vi "CML Main.vi"() -> ()   [LabVIEW 2024]
doc: "This Continuous Measurement sample project is based on the Queued Message Handler template.\n\nThe Event Handling Loop generates messages based on user interface actions.\n\nThe Message Handling Loop processes messages generated by the Event Handling Loop, or by other messages. There are also Acquisition and Logging message handling loop subVIs, and a chart updating loop."
uses:
  Settings/Settings.ctl
  Acquisition/Hardware Configuration.ctl
  Acquisition/Signal Type.ctl
  Logging/Logging Configuration.ctl
  controls/CML UI Data.ctl
  controls/CML UI State.ctl
  Logging/Logging State.ctl
  Acquisition/Acquisition State.ctl
  support/Message Queue/Enqueue Message (Single).vi
  <vilib>/Utility/error.llb/Error Cluster From Error Code.vi
  support/Message Queue/Enqueue Message (Array).vi
  <vilib>/ErrorRing/Error Ring.xnode
  Settings/CML Settings.lvlib
  Acquisition/CML Acquisition.lvlib
  Logging/CML Logging.lvlib
  support/User Event - Stop/CML User Event - Stop.lvlib
  support/Message Queue/CML Message Queue.lvlib
  Settings/Settings Dialog.vi
panel:
  out "Data":waveform(dbl)[](graph)
  in  "Settings":bool
  in  "Start":bool
  in  "Stop":bool
  out "Status":string
  in  "Exit":bool
  # "Continuous Measurement Data Logger"
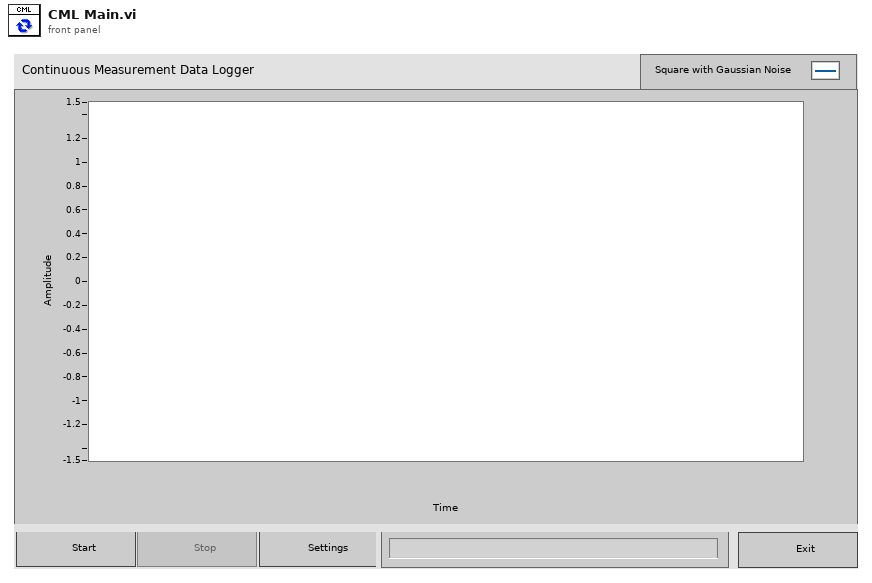
[diagram p1: front panel]
types:
  T1 = typedef "CML UI State.ctl" = enum16{"Idle", "Acquiring and Logging", "Waiting for Exit", "Waiting for Exit (Acq Stopped)", "Waiting for Exit (Log Stopped)", "Waiting for Stop", "Waiting for Stop (Acq Stopped)", "Waiting for Stop (Log Stopped)"}
  T2 = typedef "CML UI Data.ctl" = cluster{"Start Ref":refnum<vi>, "Stop Ref":refnum<vi>, "Settings Ref":refnum<vi>, "Exit Ref":refnum<vi>, "Status Ref":refnum<vi>, "Data Ref":refnum<vi>}
  T3 = typedef "CML Settings.lvlib/Settings.ctl" = cluster{"Hardware Configuration":T4, "Logging Configuration":T6}
  T4 = typedef "CML Acquisition.lvlib/Hardware Configuration.ctl" = cluster{"HW Refnum <Replace Me>":string, "Signal Type <Replace Me>":T5}
  T5 = typedef "CML Acquisition.lvlib/Signal Type.ctl" = enum16{"Sine Wave", "Square with Noise"}
  T6 = typedef "CML Logging.lvlib/Logging Configuration.ctl" = cluster{"Log File Base Path":path, "TDMS File Reference":refnum<k34>}
  T7 = typedef "CML Message Queue.lvlib/All Message Queues.ctl" = cluster{"UI":refnum<queue>, "Acquisition":refnum<queue>, "Logging":refnum<queue>}
  T8 = typedef "CML Acquisition.lvlib/Acquisition State.ctl" = enum16{"Idle", "Acquiring"}
  T9 = typedef "CML Logging.lvlib/Logging State.ctl" = enum16{"Idle", "Logging"}
  T10 = enum16{"open", "open or create", "create or replace", "create", "open (read-only)"}
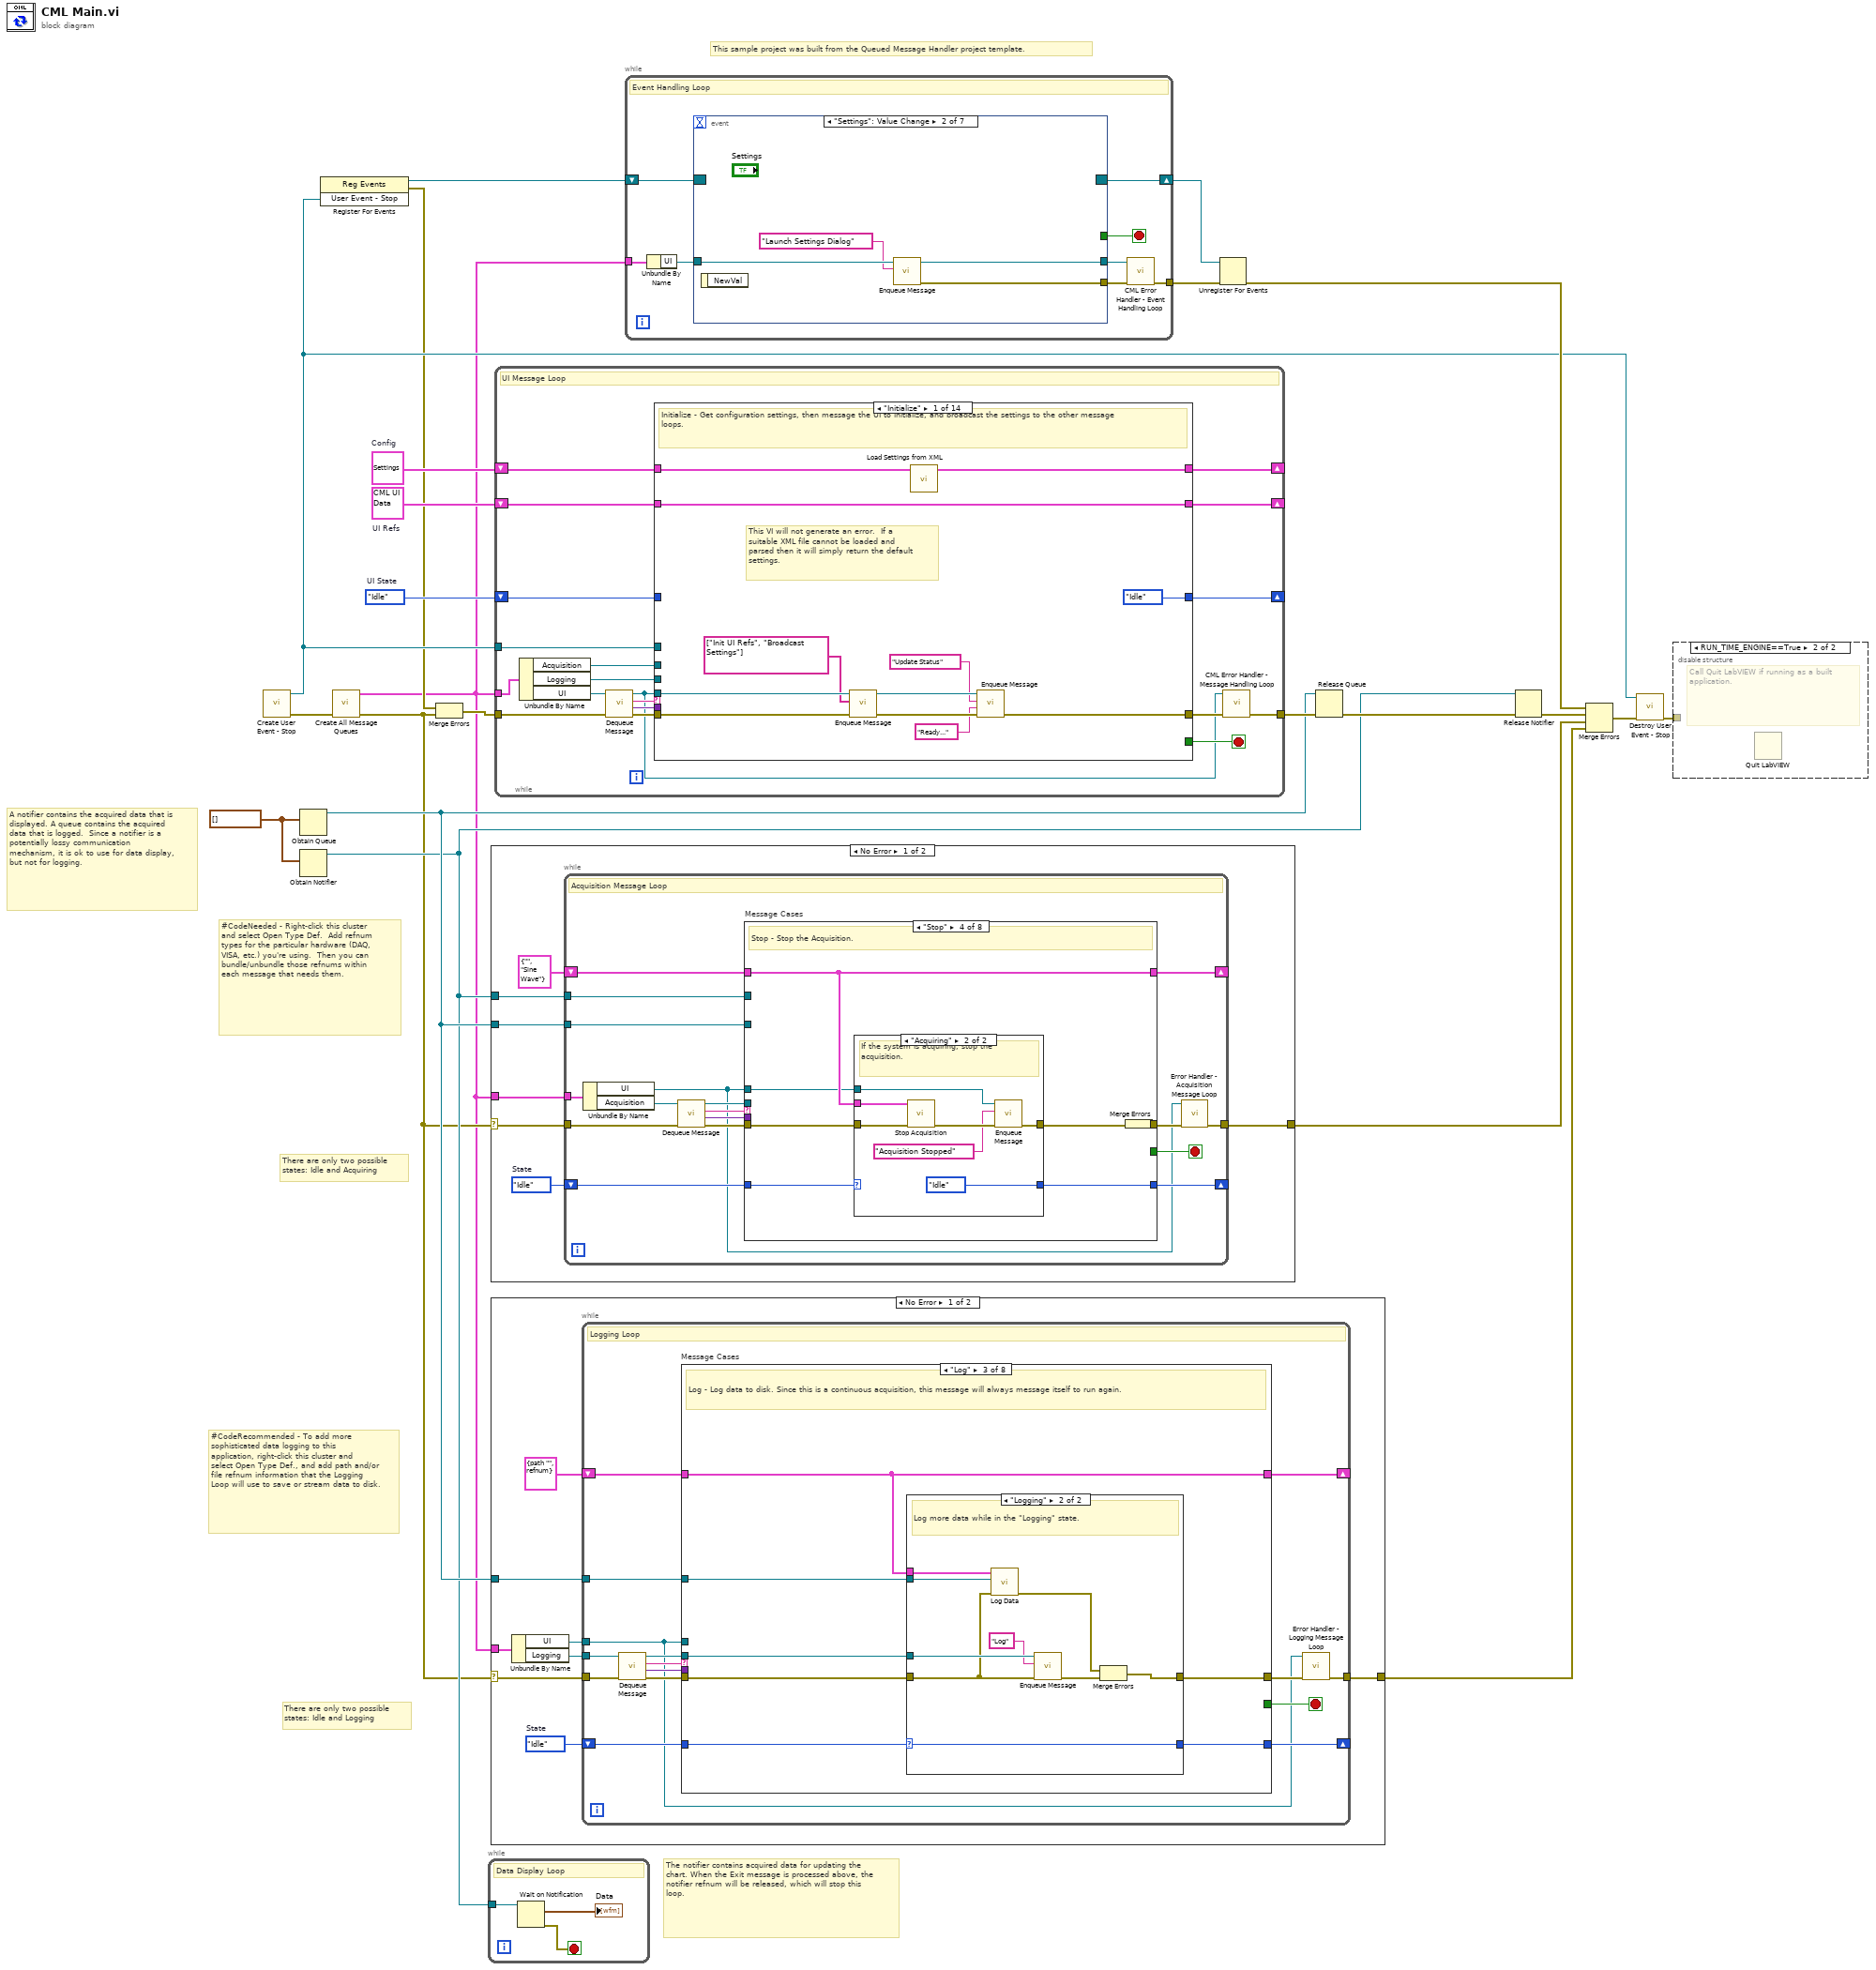
[diagram p0: block diagram]
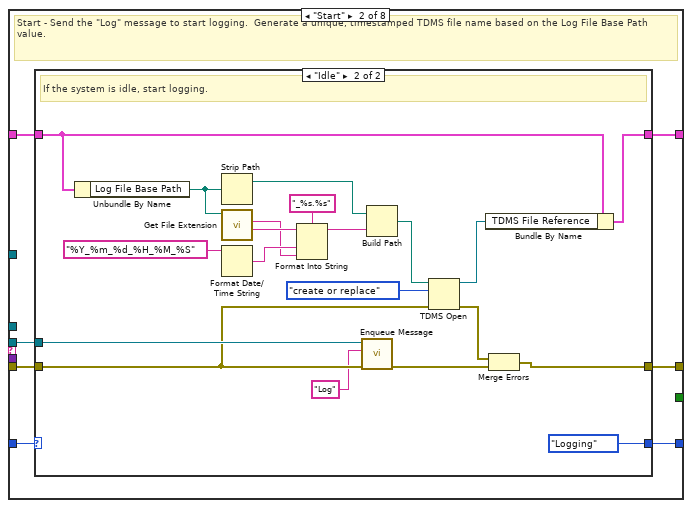
[diagram p3: hidden frame]
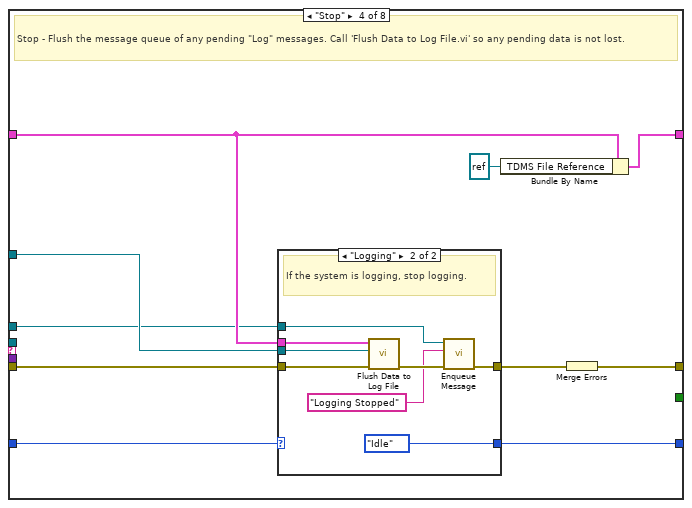
[diagram p6: hidden frame]
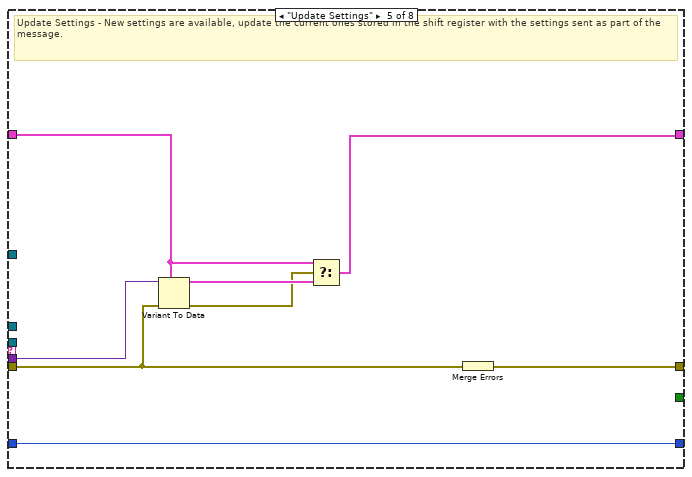
[diagram p8: hidden frame]
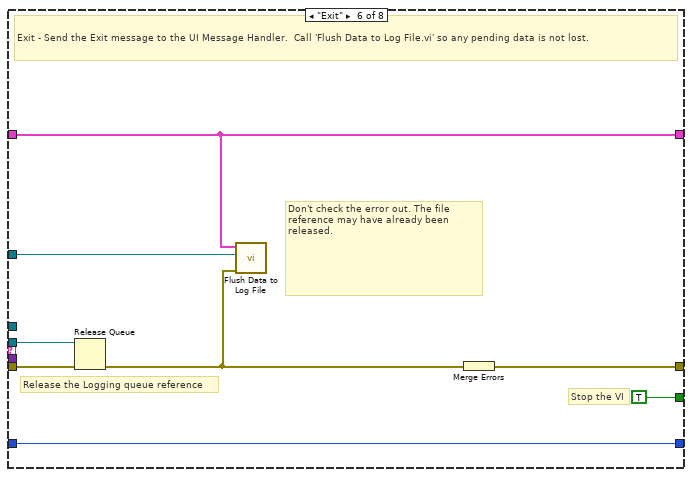
[diagram p9: hidden frame]
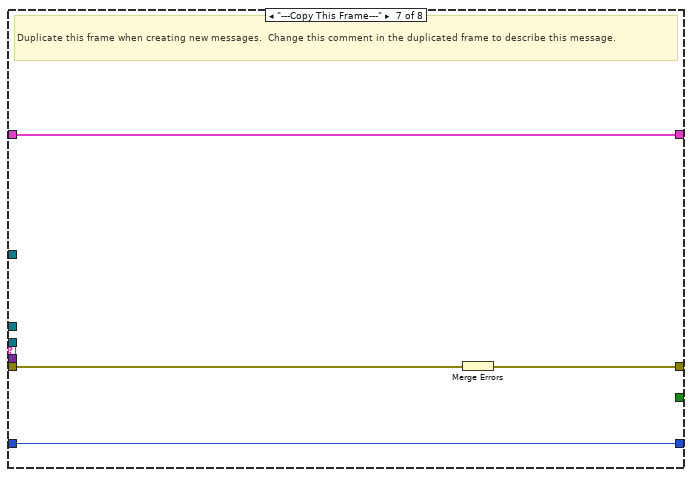
[diagram p10: hidden frame]
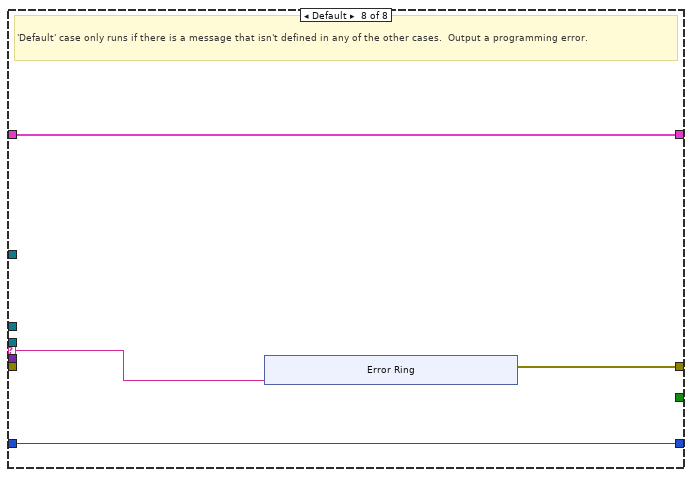
[diagram p11: hidden frame]
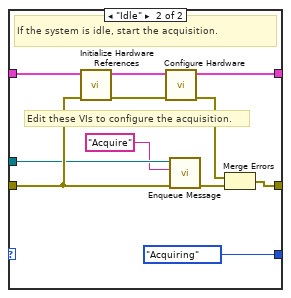
[diagram p15: hidden frame]
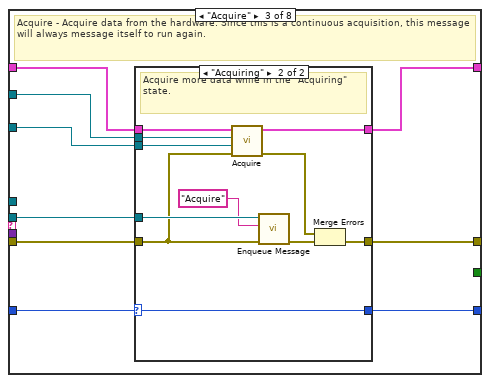
[diagram p16: hidden frame]
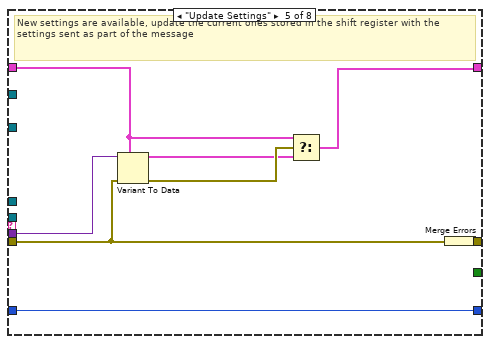
[diagram p19: hidden frame]
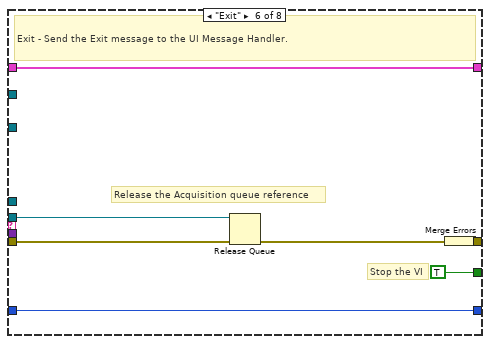
[diagram p20: hidden frame]
diagram:
  w15 = CML_UI_State."Idle"  # UI State
  w10 = waveform(dbl)[] []
  w16 = T2 {"Start Ref"=refnum, "Stop Ref"=refnum, "Settings Ref"=refnum, "Exit Ref"=refnum, "Status Ref"=refnum, "Data Ref"=refnum}  # UI Refs
  w19 = T3 {"Hardware Configuration"={"HW Refnum <Replace Me>"="", "Signal Type <Replace Me>"=enum."Sine Wave"}, "Logging Configuration"={"Log File Base Path"=path "", "TDMS File Reference"=refnum}}  # Config
  # "There are only two possible\nstates: Idle and Logging"
  # "There are only two possible\nstates: Idle and Acquiring"
  # "#CodeRecommended - To add more sophisticated data logging to this application, right-click this cluster and select Open Type Def., and add path and/or file refnum information that the Logging Loop will use to save or stream data to disk."
  # "#CodeNeeded - Right-click this cluster and select Open Type Def.  Add refnum types for the particular hardware (DAQ, VISA, etc.) you're using.  Then you can bundle/unbundle those refnums within each message that needs them."
  # "This sample project was built from the Queued Message Handler project template."
  # "A notifier contains the acquired data that is displayed. A queue contains the acquired data that is logged.  Since a notifier is a potentially lossy communication mechanism, it is ok to use for data display, but not for logging."
  # "The notifier contains acquired data for updating the chart. When the Exit message is processed above, the notifier refnum will be released, which will stop this loop."
  n1 = call "Create User Event - Stop.vi"() -> ("error out"=w20:errorcluster, "User Event - Stop"=w8:refnum<user-event>)  [unwired: 10 in]
  n2 = Obtain Queue(element data type=w10) -> (queue out=w22:refnum<queue>)  [unwired: 4 in, 2 out]
  n3 = Obtain Notifier(notification data type=w10) -> (notifier out=w5:refnum<notifier>)  [unwired: 3 in, 2 out]
  n4 = register-events(w8) -> (reference out=w9:refnum<event-registration>, error out=w6:errorcluster)  [unwired: 2 in]
  n5 = call "Create All Message Queues.vi"("error in (no error)"=w20) -> ("error out"=w3:errorcluster, "Message Queues out"=w1:T7)  [unwired: 9 in]
  n6 = Merge Errors(w6, w3) -> (w7:errorcluster)
  n7 = while "Data Display Loop" {
    tunnel: w5 -> [w26]
    stop <- w24 stop-if-true
    # "Data Display Loop"
    n8 = Wait on Notification(notifier=w26) -> (notification=→"Data":waveform(dbl)[], error out=w24:errorcluster)  [unwired: 3 in, 2 out]
  }
  n9 = case shown="No Error" w3 {
    selector: w3 -> [w31 w144]
    tunnel: w1 -> [w27 _]
    tunnel: [w33 w144] -> w4
    tunnel: w5 -> [w30 _]
    tunnel: w22 -> [w29 _]
    frame No Error {
      w28 = Acquisition_State."Idle"  # State
      n10 = while {
        shift-right: [w49] -> _
        shift-left: T4 {"HW Refnum <Replace Me>"="", "Signal Type <Replace Me>"=enum."Sine Wave"} ("Data Cluster") -> [w50]
        tunnel: w30 -> [w43]
        tunnel: w29 -> [w42]
        shift-right: [w40] -> _
        shift-left: w28 -> [w41]
        tunnel: w31 -> [w47]
        tunnel: [w39] -> w33
        tunnel: w27 -> [w36]
        stop <- w48 stop-if-true
        # "Acquisition Message Loop"
        n11 = Unbundle By Name(w36) -> ("UI"=w35:refnum<queue>, "Acquisition"=w34:refnum<queue>)
        n12 = call "Dequeue Message.vi"("error in (no error)"=w47, "Message Queue"=w34) -> ("error out"=w46:errorcluster, "Message Data"=w44:variant, "Message"=w45:string, "dup Message Queue"=w37:refnum<queue>)  [unwired: 6 in]
        n13 = case "Message Cases" shown="\"Stop\"" w45 {
          selector: w45 -> [_ _ _ _ _ _ _ w133]
          tunnel: w37 -> [_ w57 w82 _ _ w123 _ _]
          tunnel: w46 -> [w53 w58 w81 w103 w115 w125 w132 _]
          tunnel: [w53 w60 w83 w104 w121 w127 w130 w134] -> w38
          tunnel: w50 -> [w52 w59 w79 w101 w117 w126 w131 w136]
          tunnel: [w52 w56 w80 w101 w116 w126 w131 w136] -> w49
          tunnel: [_ _ _ _ _ TRUE _ _] -> w48
          tunnel: w44 -> [_ _ _ _ w120 _ _ _]
          tunnel: w35 -> [_ _ _ w98 _ _ _ _]
          tunnel: w43 -> [_ _ w78 _ _ _ _ _]
          tunnel: w42 -> [_ _ w77 _ _ _ _ _]
          tunnel: w41 -> [w51 w54 w75 w100 w114 w122 w129 w135]
          tunnel: [w51 w55 w76 w99 w114 w122 w129 w135] -> w40
          frame "Initialize" {
            # "Initialize  - Initialize is currently a no-op.  The hardware initialization takes place in the 'Start' message."
          }
          frame "Start" {
            # "Start - Configure and start the acquisition."
            n14 = case shown="\"Acquiring\"" w54 {
              selector: w54 -> [w61 _]
              tunnel: [w62 w74] -> w60
              tunnel: w59 -> [w63 w73]
              tunnel: w58 -> [w62 w72]
              tunnel: w57 -> [_ w70]
              tunnel: [w63 w66] -> w56
              tunnel: [w61 Acquisition_State."Acquiring" ("Acquisition State")] -> w55
              frame "Acquiring" {
                # "The system is already acquiring. Ignore the \"Start\" message."
              }
              frame "Idle" {
                # "Edit these VIs to configure the acquisition."
                # "If the system is idle, start the acquisition."
                n15 = call "Initialize Hardware References.vi"("error in (no error)"=w72, "Hardware Resources in"=w73) -> ("error out"=w69:errorcluster, "Hardware Resources out"=w67:T4)  [unwired: 8 in]
                n16 = call "Configure Hardware.vi"("error in (no error)"=w69, "Hardware Resources in"=w67) -> ("error out"=w68:errorcluster, "Hardware Resources out"=w66:T4)  [unwired: 8 in]
                n17 = call-poly "Enqueue Message.vi"("error in (no error)"=w72, "Message"="Acquire", "Message Queue"=w70) -> ("error out"=w71:errorcluster)  [unwired: 7 in, 1 out]
                n18 = Merge Errors(w68, w71) -> (w74:errorcluster)
              }
            }
          }
          frame "Acquire" {
            # "Acquire - Acquire data from the hardware. Since this is a continuous acquisition, this message will always message itself to run again."
            n19 = case shown="\"Acquiring\"" w75 {
              selector: w75 -> [w84 w88]
              tunnel: [w85 w97] -> w83
              tunnel: w82 -> [_ w95]
              tunnel: w81 -> [w85 w87]
              tunnel: [w86 w93] -> w80
              tunnel: w79 -> [w86 w92]
              tunnel: w78 -> [_ w90]
              tunnel: w77 -> [_ w89]
              tunnel: [w84 w88] -> w76
              frame "Idle" {
                # "Ignore \"Acquire\" messages when the acquisition is idle."
              }
              frame "Acquiring" {
                # "Acquire more data while in the \"Acquiring\" state."
                n20 = call "Acquire.vi"("error in (no error)"=w87, "Data Queue"=w89, "Data Notifier"=w90, "Hardware Resources in"=w92) -> ("error out"=w94:errorcluster, "Hardware Resources out"=w93:T4)  [unwired: 6 in]
                n21 = call-poly "Enqueue Message.vi"("error in (no error)"=w87, "Message"="Acquire", "Message Queue"=w95) -> ("error out"=w96:errorcluster)  [unwired: 7 in, 1 out]
                n22 = Merge Errors(w94, w96) -> (w97:errorcluster)
              }
            }
          }
          frame "Stop" {
            # "Stop - Stop the Acquisition."
            n23 = case shown="\"Acquiring\"" w100 {
              selector: w100 -> [w105 _]
              tunnel: w103 -> [w106 w113]
              tunnel: [w106 w109] -> w102
              tunnel: w101 -> [_ w111]
              tunnel: [w105 Acquisition_State."Idle" ("State")] -> w99
              tunnel: w98 -> [_ w108]
              frame "Idle" {
                # "The system is already idle. Ignore the \"Stop\" message."
              }
              frame "Acquiring" {
                # "If the system is acquiring, stop the acquisition."
                n24 = call "Stop Acquisition.vi"("error in (no error)"=w113, "Hardware Resources in"=w111) -> ("error out"=w112:errorcluster)  [unwired: 9 in]
                n25 = call-poly "Enqueue Message.vi"("error in (no error)"=w112, "Message"="Acquisition Stopped", "Message Queue"=w108) -> ("error out"=w109:errorcluster)  [unwired: 7 in, 1 out]
              }
            }
            n26 = Merge Errors(w102) -> (w104:errorcluster)
          }
          frame "Update Settings" {
            # "New settings are available, update the current ones stored in the shift register with the settings sent as part of the message"
            n27 = Variant To Data(error in=w115, type=w117, Variant=w120) -> (data=w118:T4, error out=w119:errorcluster)
            n28 = Select(t=w117, s=w119, f=w118) -> (s? t:f=w116:T4)
            n29 = Merge Errors(w115) -> (w121:errorcluster)
          }
          frame "Exit" {
            # "Release the Acquisition queue reference"
            # "Stop the VI"
            # "Exit - Send the Exit message to the UI Message Handler."
            n30 = Release Queue(queue=w123, error in (no error)=w125) -> (error out=w124:errorcluster)  [unwired: 1 in, 2 out]
            n31 = Merge Errors(w124) -> (w127:errorcluster)
          }
          frame "---Copy This Frame---" {
            # "Duplicate this frame when creating new messages.  Change this comment in the duplicated frame to describe this message."
            n32 = Merge Errors(w132) -> (w130:errorcluster)
          }
          frame Default {
            # "'Default' case only runs if there is a message that isn't defined in any of the other cases.  Output a programming error."
            n33 = xnode "Error Ring"("parameter 0"=w133) -> ("error out"=w134:errorcluster)
          }
        }
        n34 = call "Error Handler - Acquisition Message Loop.vi"("error in (no error)"=w38, "Message Queue"=w35) -> ("dup error in"=w39:errorcluster)  [unwired: 8 in, 1 out]
      }
    }
    frame Error {
    }
  }
  n35 = case shown="No Error" w3 {
    selector: w3 -> [w148 w270]
    tunnel: w1 -> [w152 _]
    tunnel: [w150 w270] -> w2
    tunnel: w22 -> [w147 _]
    frame No Error {
      w145 = Logging_State."Idle"  # State
      n36 = Unbundle By Name(w152) -> ("UI"=w146:refnum<queue>, "Logging"=w151:refnum<queue>)
      n37 = while {
        tunnel: w151 -> [w159]
        shift-right: [w166] -> _
        shift-left: T6 {"Log File Base Path"=path "", "TDMS File Reference"=refnum} ("Logging Configuration") -> [w167]
        tunnel: w146 -> [w153]
        tunnel: w147 -> [w158]
        shift-right: [w156] -> _
        shift-left: w145 -> [w157]
        tunnel: w148 -> [w164]
        tunnel: [w155] -> w150
        stop <- w165 stop-if-true
        # "Logging Loop"
        n38 = call "Dequeue Message.vi"("error in (no error)"=w164, "Message Queue"=w159) -> ("error out"=w163:errorcluster, "Message Data"=w161:variant, "Message"=w162:string, "dup Message Queue"=w160:refnum<queue>)  [unwired: 6 in]
        n39 = case "Message Cases" shown="\"Log\"" w162 {
          selector: w162 -> [_ _ _ _ _ _ _ w259]
          tunnel: w160 -> [_ w176 w206 _ _ w251 _ _]
          tunnel: w163 -> [w169 w175 w204 w222 w240 w252 w258 _]
          tunnel: [w169 w177 w207 w228 w246 w253 w256 w260] -> w154
          tunnel: w167 -> [w170 w174 w203 w223 w244 w249 w257 w262]
          tunnel: [w170 w173 w203 w226 w241 w249 w257 w262] -> w166
          tunnel: [_ _ _ _ _ TRUE _ _] -> w165
          tunnel: w161 -> [_ _ _ _ w245 _ _ _]
          tunnel: w153 -> [_ _ _ w219 _ _ _ _]
          tunnel: w158 -> [_ _ w205 w224 _ w248 _ _]
          tunnel: w157 -> [w168 w172 w202 w221 w239 w247 w255 w261]
          tunnel: [w168 w171 w201 w220 w239 w247 w255 w261] -> w156
          frame "Initialize" {
            # "Initialize - gets called when first launched. Currently a no-op."
          }
          frame "Start" {
            # "Start - Send the \"Log\" message to start logging.  Generate a unique, timestamped TDMS file name based on the Log File Base Path value."
            n40 = case shown="\"Idle\"" w172 {
              selector: w172 -> [w179 _]
              tunnel: [w178 w183] -> w177
              tunnel: w176 -> [_ w184]
              tunnel: w175 -> [w178 w182]
              tunnel: w174 -> [w180 w185]
              tunnel: [w180 w187] -> w173
              tunnel: [w179 Logging_State."Logging" ("State")] -> w171
              frame "Logging" {
                # "The system is already logging. Ignore the \"Start\" message."
              }
              frame "Idle" {
                # "If the system is idle, start logging."
                n41 = Unbundle By Name(w185) -> ("Log File Base Path"=w200:path)
                n42 = Strip Path(path=w200) -> (stripped path=w197:path)  [unwired: 1 out]
                n43 = call <vilib>:"Get File Extension.vi"("file"=w200) -> ("filename without extension"=w198:string, "lowercase file extension"=w194:string)  [unwired: 6 in, 3 out]
                n44 = Format Date/Time String(time format string (%c)="%Y_%m_%d_%H_%M_%S") -> (date/time string=w195:string)  [unwired: 2 in]
                n45 = Format Into String(format string="_%s.%s", initial string=w198, w195, w194) -> (resulting string=w193:string)  [unwired: 1 in, 1 out]
                n46 = call-poly "Enqueue Message.vi"("error in (no error)"=w182, "Message"="Log", "Message Queue"=w184) -> ("error out"=w190:errorcluster)  [unwired: 7 in, 1 out]
                n47 = Build Path(base path=w197, name or relative path=w193) -> (appended path=w192:path)
                n48 = TDMS Open(8:w182, 10:T10."create or replace" ("operation (0:open)"), 11:w192) -> (0:w191:errorcluster, 3:w188:refnum<k34>)  [unwired: 4 in]
                n49 = Bundle By Name(cluster=w185, "TDMS File Reference"=w188) -> (w187:T6)
                n50 = Merge Errors(w191, w190) -> (w183:errorcluster)
              }
            }
          }
          frame "Log" {
            # "Log - Log data to disk. Since this is a continuous acquisition, this message will always message itself to run again."
            n51 = case shown="\"Logging\"" w202 {
              selector: w202 -> [w209 w211]
              tunnel: [w208 w218] -> w207
              tunnel: w206 -> [_ w216]
              tunnel: w205 -> [_ w215]
              tunnel: w204 -> [w208 w210]
              tunnel: w203 -> [_ w212]
              tunnel: [w209 w211] -> w201
              frame "Idle" {
                # "Ignore \"Log\" messages when the logging is idle."
              }
              frame "Logging" {
                # "Log more data while in the \"Logging\" state."
                n52 = call "Log Data.vi"("error in (no error)"=w210, "Data Queue"=w215, "Logging Configuration"=w212) -> ("error out"=w214:errorcluster)  [unwired: 8 in]
                n53 = call-poly "Enqueue Message.vi"("error in (no error)"=w210, "Message"="Log", "Message Queue"=w216) -> ("error out"=w217:errorcluster)  [unwired: 7 in, 1 out]
                n54 = Merge Errors(w214, w217) -> (w218:errorcluster)
              }
            }
          }
          frame "Stop" {
            # "Stop - Flush the message queue of any pending \"Log\" messages. Call 'Flush Data to Log File.vi' so any pending data is not lost."
            n55 = case shown="\"Logging\"" w221 {
              selector: w221 -> [w229 _]
              tunnel: [w230 w233] -> w227
              tunnel: w224 -> [_ w237]
              tunnel: w223 -> [_ w236]
              tunnel: w222 -> [w230 w235]
              tunnel: [w229 Logging_State."Idle" ("State")] -> w220
              tunnel: w219 -> [_ w232]
              frame "Idle" {
                # "The system is already idle. Ignore the \"Stop\" message."
              }
              frame "Logging" {
                # "If the system is logging, stop logging."
                n56 = call "Flush Data to Log File.vi"("error in (no error)"=w235, "Data Queue"=w237, "Logging Configuration"=w236) -> ("error out"=w238:errorcluster)  [unwired: 8 in]
                n57 = call-poly "Enqueue Message.vi"("error in (no error)"=w238, "Message"="Logging Stopped", "Message Queue"=w232) -> ("error out"=w233:errorcluster)  [unwired: 7 in, 1 out]
              }
            }
            n58 = Bundle By Name(cluster=w223, "TDMS File Reference"=refnum<k34> refnum) -> (w226:T6)
            n59 = Merge Errors(w227) -> (w228:errorcluster)
          }
          frame "Update Settings" {
            # "Update Settings - New settings are available, update the current ones stored in the shift register with the settings sent as part of the message."
            n60 = Variant To Data(error in=w240, type=w244, Variant=w245) -> (data=w243:T6, error out=w242:errorcluster)
            n61 = Select(t=w244, s=w242, f=w243) -> (s? t:f=w241:T6)
            n62 = Merge Errors(w240) -> (w246:errorcluster)
          }
          frame "Exit" {
            # "Don't check the error out. The file reference may have already been released."
            # "Release the Logging queue reference"
            # "Stop the VI"
            # "Exit - Send the Exit message to the UI Message Handler.  Call 'Flush Data to Log File.vi' so any pending data is not lost."
            n63 = Release Queue(queue=w251, error in (no error)=w252) -> (error out=w250:errorcluster)  [unwired: 1 in, 2 out]
            n64 = call "Flush Data to Log File.vi"("error in (no error)"=w250, "Data Queue"=w248, "Logging Configuration"=w249) -> ()  [unwired: 8 in, 1 out]
            n65 = Merge Errors(w250) -> (w253:errorcluster)
          }
          frame "---Copy This Frame---" {
            # "Duplicate this frame when creating new messages.  Change this comment in the duplicated frame to describe this message."
            n66 = Merge Errors(w258) -> (w256:errorcluster)
          }
          frame Default {
            # "'Default' case only runs if there is a message that isn't defined in any of the other cases.  Output a programming error."
            n67 = xnode "Error Ring"("parameter 0"=w259) -> ("error out"=w260:errorcluster)
          }
        }
        n68 = call "Error Handler - Logging Message Loop.vi"("error in (no error)"=w154, "Message Queue"=w153) -> ("dup error in"=w155:errorcluster)  [unwired: 8 in, 1 out]
      }
    }
    frame Error {
    }
  }
  n69 = while {
    tunnel: w8 -> [w288]
    shift-right: [w283] -> _
    shift-left: w19 -> [w282]
    shift-right: [w280] -> _
    shift-left: w16 -> [w281]
    shift-right: [w275] -> _
    shift-left: w15 -> [w276]
    tunnel: w7 -> [w287]
    tunnel: [w279] -> w23
    tunnel: w1 -> [w274]
    stop <- w289 stop-if-true
    # "UI Message Loop"
    n70 = Unbundle By Name(w274) -> ("Acquisition"=w271:refnum<queue>, "Logging"=w272:refnum<queue>, "UI"=w273:refnum<queue>)
    n71 = call "Dequeue Message.vi"("error in (no error)"=w287, "Message Queue"=w273) -> ("error out"=w286:errorcluster, "Message Data"=w284:variant, "Message"=w285:string, "dup Message Queue"=w277:refnum<queue>)  [unwired: 6 in]
    n72 = case "Message Cases" shown="\"Initialize\"" w285 {
      selector: w285 -> [_ _ _ _ _ _ _ _ _ _ _ _ _ w507]
      tunnel: w277 -> [w293 _ _ w346 _ w371 w396 _ w436 _ w457 w483 _ _]
      tunnel: w286 -> [w292 w315 w324 w345 w365 w372 w397 w424 w438 w445 w456 w499 w505 _]
      tunnel: [w297 w315 w325 w330 w366 w369 w394 w429 w431 w448 w455 w485 w504 w506] -> w278
      tunnel: [_ _ _ _ _ _ _ _ _ _ _ TRUE _ _] -> w289
      tunnel: w284 -> [_ _ w323 _ _ _ _ _ _ w449 _ w482 _ _]
      tunnel: w288 -> [_ _ _ _ _ _ _ _ _ _ _ w497 _ _]
      tunnel: [w300 w314 w319 w344 w364 w375 w400 w427 w435 w453 w460 w495 w503 w510] -> w283
      tunnel: w282 -> [w301 w314 w319 w344 w364 w375 w400 w427 w439 w453 w460 w495 w503 w510]
      tunnel: w281 -> [w294 w313 w318 w342 w363 w374 w399 w423 w433 w452 w459 w494 w502 w509]
      tunnel: [w294 w310 w318 w342 w363 w374 w399 w423 w433 w452 w459 w494 w502 w509] -> w280
      tunnel: w271 -> [_ _ _ w329 w350 _ _ w430 _ _ _ w493 _ _]
      tunnel: w272 -> [_ _ _ w332 w353 _ _ w422 _ _ _ w492 _ _]
      tunnel: w276 -> [_ _ w317 _ w347 w373 w398 w421 w432 w447 w458 _ w501 w508]
      tunnel: [CML_UI_State."Idle" ("UI State") CML_UI_State."Idle" ("UI State") w317 CML_UI_State."Acquiring and Logging" ("UI State") w348 w370 w395 w421 w432 w447 w454 CML_UI_State."Idle" ("UI State") w501 w508] -> w275
      frame "Initialize" {
        # "This VI will not generate an error.  If a suitable XML file cannot be loaded and parsed then it will simply return the default settings."
        # "Initialize - Get configuration settings, then message the UI to initialize, and broadcast the settings to the other message loops."
        n73 = call-poly "Enqueue Message.vi"("error in (no error)"=w292, "Message Array"=string[] ["Init UI Refs", "Broadcast Settings"], "Message Queue"=w293) -> ("error out"=w299:errorcluster, "dup Message Queue"=w298:refnum<queue>)  [unwired: 7 in]
        n74 = call "Load Settings from XML.vi"("Settings in"=w301) -> ("Settings out"=w300:T3)  [unwired: 9 in, 1 out]
        n75 = call-poly "Enqueue Message.vi"("error in (no error)"=w299, "Message Data"="Ready..." ("Ready..."), "Message"="Update Status", "Message Queue"=w298) -> ("error out"=w297:errorcluster)  [unwired: 6 in, 1 out]
      }
      frame "Init UI Refs" {
        # "Enable: Start, Exit, Settings\nDisable: Stop"
        # "Init UI Refs - Store control references for UI controls.  Also enable/disable controls appropriately."
        n76 = control-ref of="Data"() -> (w311:refnum<vi>)
        n77 = control-ref of="Start"() -> (w305:refnum<vi>)
        n78 = control-ref of="Stop"() -> (w316:refnum<vi>)
        n79 = control-ref of="Settings"() -> (w304:refnum<vi>)
        n80 = control-ref of="Exit"() -> (w303:refnum<vi>)
        n81 = control-ref of="Status"() -> (w312:refnum<vi>)
        n82 = Bundle By Name(cluster=w313, "Start Ref"=w305, "Stop Ref"=w316, "Settings Ref"=w304, "Exit Ref"=w303, "Status Ref"=w312, "Data Ref"=w311) -> (w310:T2)
        n83 = Build Array(w305, w304, w303) -> (w308:refnum<vi>[])
        n84 = Build Array(w316) -> (w307:refnum<vi>[])
        n85 = call "CML Set Enable State on Multiple Controls.vi"("Enable?"=TRUE, "Controls"=w308) -> ()  [unwired: 10 in]
        n86 = call "CML Set Enable State on Multiple Controls.vi"("Enable?"=FALSE, "Controls"=w307) -> ()  [unwired: 10 in]
      }
      frame "Update Status" {
        # "Update Status - Convert the message data to a string to display in the Status indicator."
        n87 = Variant To Data(error in=w324, type="", Variant=w323) -> (data=→"Status":string, error out=w321:errorcluster)
        n88 = Merge Errors(w321) -> (w325:errorcluster)
      }
      frame "Start" {
        w326 = "Start" ("Message")
        # "Message Acquisition and Logging loops to start."
        # "Enable: Stop\n\nDisable: Start, Exit, Settings"
        # "Start - Enable/Disable buttons appropriately for an acquisition that has started, and update status display."
        n89 = Unbundle By Name(w342) -> ("Stop Ref"=w337:refnum<vi>, "Start Ref"=w336:refnum<vi>, "Exit Ref"=w335:refnum<vi>, "Settings Ref"=w334:refnum<vi>)
        n90 = call-poly "Enqueue Message.vi"("error in (no error)"=w345, "Message Data"="Acquiring and Logging..." ("Acquiring and Logging..."), "Message"="Update Status", "Message Queue"=w346) -> ("error out"=w333:errorcluster)  [unwired: 6 in, 1 out]
        n91 = Build Array(w336, w335, w334) -> (w340:refnum<vi>[])
        n92 = Build Array(w337) -> (w339:refnum<vi>[])
        n93 = call "CML Set Enable State on Multiple Controls.vi"("Enable?"=TRUE, "Controls"=w339) -> ()  [unwired: 10 in]
        n94 = call "CML Set Enable State on Multiple Controls.vi"("Enable?"=FALSE, "Controls"=w340) -> ()  [unwired: 10 in]
        n95 = call-poly "Enqueue Message.vi"("error in (no error)"=w333, "Message"=w326, "Message Queue"=w332) -> ("error out"=w331:errorcluster)  [unwired: 7 in, 1 out]
        n96 = call-poly "Enqueue Message.vi"("error in (no error)"=w331, "Message"=w326, "Message Queue"=w329) -> ("error out"=w330:errorcluster)  [unwired: 7 in, 1 out]
      }
      frame "Stop" {
        # "Message Acquisition and Logging loops to stop"
        # "Enable: Start, Exit, Settings\nDisable: Stop"
        # "Stop - Enable/Disable buttons appropriately for an acquisition that has stopped, and update status display."
        n97 = Unbundle By Name(w363) -> ("Stop Ref"=w358:refnum<vi>, "Start Ref"=w357:refnum<vi>, "Exit Ref"=w356:refnum<vi>, "Settings Ref"=w355:refnum<vi>)
        n98 = Build Array(w357, w356, w355) -> (w361:refnum<vi>[])
        n99 = Build Array(w358) -> (w360:refnum<vi>[])
        n100 = call "CML Set Enable State on Multiple Controls.vi"("Enable?"=FALSE, "Controls"=w360) -> ()  [unwired: 10 in]
        n101 = call "CML Set Enable State on Multiple Controls.vi"("Enable?"=TRUE, "Controls"=w361) -> ()  [unwired: 10 in]
        n102 = call-poly "Enqueue Message.vi"("error in (no error)"=w365, "Message"="Stop", "Message Queue"=w353) -> ("error out"=w352:errorcluster)  [unwired: 7 in, 1 out]
        n103 = case shown="Default" w347 {
          selector: w347 -> [w367 _]
          tunnel: [w367 CML_UI_State."Waiting for Stop" ("UI State")] -> w348
          frame "Waiting for Exit" {
          }
          frame Default {
          }
        }
        n104 = call-poly "Enqueue Message.vi"("error in (no error)"=w352, "Message"="Stop", "Message Queue"=w350) -> ("error out"=w351:errorcluster)  [unwired: 7 in, 1 out]
        n105 = Merge Errors(w351) -> (w366:errorcluster)
      }
      frame "Acquisition Stopped" {
        # "Logic for determining what action to take when the acquisition has stopped."
        n106 = case shown="\"Waiting for Stop\", \"Waiting for Stop (Acq Stopped)\"" w373 {
          selector: w373 -> [w377 _ _ _ _]
          tunnel: w372 -> [w376 w379 w381 w387 w393]
          tunnel: w371 -> [_ _ _ w385 w390]
          tunnel: [w377 CML_UI_State."Waiting for Exit (Acq Stopped)" ("UI State") CML_UI_State."Waiting for Stop (Acq Stopped)" ("UI State") CML_UI_State."Idle" ("UI State") CML_UI_State."Idle" ("UI State")] -> w370
          tunnel: [w376 w379 w381 w386 w391] -> w369
          frame Default {
          }
          frame "Waiting for Exit", "Waiting for Exit (Acq Stopped)" {
          }
          frame "Waiting for Stop", "Waiting for Stop (Acq Stopped)" {
          }
          frame "Waiting for Exit (Log Stopped)" {
            # "If we are waiting to exit, and the logging has already stopped, then the \"Acquisition Stopped\" message indicates that it is time to exit."
            n107 = call-poly "Enqueue Message.vi"("Priority Message? (F)"=TRUE, "error in (no error)"=w387, "Message"="Exit", "Message Queue"=w385) -> ("error out"=w386:errorcluster)  [unwired: 6 in, 1 out]
          }
          frame "Waiting for Stop (Log Stopped)" {
            # "If we are waiting to stop, and the logging has already stopped, then the \"Acquisition Stopped\" message indicates that it is time to stop."
            n108 = call-poly "Enqueue Message.vi"("error in (no error)"=w393, "Message Data"="Ready..." ("Ready..."), "Message"="Update Status", "Message Queue"=w390) -> ("error out"=w391:errorcluster)  [unwired: 6 in, 1 out]
          }
        }
      }
      frame "Logging Stopped" {
        # "Logic for determining what action to take when the logging has stopped."
        n109 = case shown="\"Waiting for Stop (Acq Stopped)\"" w398 {
          selector: w398 -> [w402 _ _ _ _]
          tunnel: w397 -> [w401 w404 w406 w412 w417]
          tunnel: w396 -> [_ _ _ w410 w416]
          tunnel: [w402 CML_UI_State."Waiting for Exit (Log Stopped)" ("UI State") CML_UI_State."Waiting for Stop (Log Stopped)" ("UI State") CML_UI_State."Idle" ("UI State") CML_UI_State."Idle" ("UI State")] -> w395
          tunnel: [w401 w404 w406 w411 w415] -> w394
          frame Default {
          }
          frame "Waiting for Exit", "Waiting for Exit (Log Stopped)" {
          }
          frame "Waiting for Stop", "Waiting for Stop (Log Stopped)" {
          }
          frame "Waiting for Exit (Acq Stopped)" {
            # "If we are waiting to exit, and the acquisition has already stopped, then the \"Logging Stopped\" message indicates that it is time to exit."
            n110 = call-poly "Enqueue Message.vi"("Priority Message? (F)"=TRUE, "error in (no error)"=w412, "Message"="Exit", "Message Queue"=w410) -> ("error out"=w411:errorcluster)  [unwired: 6 in, 1 out]
          }
          frame "Waiting for Stop (Acq Stopped)" {
            # "If we are waiting to stop, and the acquisition has already stopped, then the \"Logging Stopped\" message indicates that it is time to stop."
            n111 = call-poly "Enqueue Message.vi"("error in (no error)"=w417, "Message Data"="Ready..." ("Ready..."), "Message"="Update Status", "Message Queue"=w416) -> ("error out"=w415:errorcluster)  [unwired: 6 in, 1 out]
          }
        }
      }
      frame "Broadcast settings" {
        w419 = "Update Settings" ("Message")
        # "Broadcast settings - Send the 'Update Settings' message to the Logging and Acquisition message loops."
        n112 = Unbundle By Name(w427) -> ("Hardware Configuration"=w426:T4, "Logging Configuration"=w420:T6)
        n113 = call-poly "Enqueue Message.vi"("Message Data"=w426, "Message"=w419, "Message Queue"=w430) -> ("error out"=w428:errorcluster)  [unwired: 7 in, 1 out]
        n114 = call-poly "Enqueue Message.vi"("error in (no error)"=w428, "Message Data"=w420, "Message"=w419, "Message Queue"=w422) -> ("error out"=w425:errorcluster)  [unwired: 6 in, 1 out]
        n115 = Merge Errors(w425, w424) -> (w429:errorcluster)
      }
      frame "Launch Settings Dialog" {
        # "Launch Settings Dialog - Launch the Settings Dialog when the user clicks the 'Settings' button."
        n116 = call-by-ref "Call By Reference"("error in (no error)"=w438, "Settings in"=w439) -> ("error out"=w434:errorcluster, "Cancelled?"=w437:bool, "Settings out"=w435:T3)  [unwired: 8 in, 3 out]
        n117 = case shown="False" w437 {
          tunnel: w436 -> [w443 _]
          tunnel: w434 -> [w442 w444]
          tunnel: [w441 w444] -> w431
          frame False {
            n118 = call-poly "Enqueue Message.vi"("error in (no error)"=w442, "Message"="Broadcast Settings", "Message Queue"=w443) -> ("error out"=w441:errorcluster)  [unwired: 7 in, 1 out]
          }
          frame True {
          }
        }
      }
      frame "Error" {
        # "Error - Display an error dialog. This message is sent by the \"Error Handler\" VIs at the end of other loops in this application."
        n119 = Variant To Data(error in=w445, type=errorcluster {"status"=FALSE, "code"=0, "source"=""} ("error constant"), Variant=w449) -> (data=w446:errorcluster, error out=w450:errorcluster)
        n120 = call <vilib>:"Simple Error Handler.vi"("error in (no error)"=w446) -> ()  [unwired: 4 in, 5 out]
        n121 = Merge Errors(w450) -> (w448:errorcluster)
      }
      frame "Confirm Quit" {
        # "Confirm Quit - Message that can confirm whether or not the user wants to exit the application."
        n122 = case shown="\"Acquiring and Logging\"" w458 {
          tunnel: w457 -> [w466 w470]
          tunnel: w456 -> [w465 w469]
          tunnel: [w464 w468] -> w455
          tunnel: [CML_UI_State."Idle" ("UI State") w467] -> w454
          frame Default {
            # "If 'Confirm Quit' comes in while the system is idle, there is no need for a confirmation message."
            n123 = call-poly "Enqueue Message.vi"("Priority Message? (F)"=TRUE, "error in (no error)"=w465, "Message"="Exit", "Message Queue"=w466) -> ("error out"=w464:errorcluster)  [unwired: 6 in, 1 out]
          }
          frame "Acquiring and Logging" {
            n124 = Two Button Dialog(message="Are you sure you want to quit while the acquisition is running?" ("Confirm Quit Message"), 1:"No" ("No"), 2:"Yes" ("Yes")) -> (T button?=w471:bool)
            n125 = case shown="True" w471 {
              tunnel: w470 -> [_ w480]
              tunnel: w469 -> [w476 w481]
              tunnel: [w476 w479] -> w468
              tunnel: [CML_UI_State."Acquiring and Logging" ("UI State") CML_UI_State."Waiting for Exit" ("UI State")] -> w467
              frame False {
                # "User did not want to quit."
              }
              frame True {
                n126 = call-poly "Enqueue Message.vi"("error in (no error)"=w481, "Message"="Stop", "Message Queue"=w480) -> ("error out"=w479:errorcluster)  [unwired: 7 in, 1 out]
              }
            }
          }
        }
      }
      frame "Exit" {
        w488 = TRUE ("Priority Message? (F)")
        w489 = "Exit" ("Message")
        # "Popup an error dialog if 'Exit' was called as a result of an error."
        # "Stop the VI"
        # "Exit - Send Exit messages to the Acquisition and Logging loops, and fire the user event to stop the Event Handling Loop."
        n127 = Variant To Data(type=errorcluster {"status"=FALSE, "code"=0, "source"=""} ("error constant"), Variant=w482) -> (data=w486:errorcluster)  [unwired: 1 in, 1 out]
        n128 = call <vilib>:"Simple Error Handler.vi"("error in (no error)"=w486) -> ()  [unwired: 4 in, 5 out]
        n129 = call-poly "Enqueue Message.vi"("Priority Message? (F)"=w488, "Message"=w489, "Message Queue"=w493) -> ("error out"=w490:errorcluster)  [unwired: 7 in, 1 out]
        n130 = Release Queue(queue=w483, error in (no error)=w499) -> (error out=w484:errorcluster)  [unwired: 1 in, 2 out]
        n131 = call-poly "Enqueue Message.vi"("Priority Message? (F)"=w488, "error in (no error)"=w490, "Message"=w489, "Message Queue"=w492) -> ("error out"=w500:errorcluster)  [unwired: 6 in, 1 out]
        n132 = call "Fire User Event - Stop.vi"("User Event - Stop"=w497) -> ("error out"=w496:errorcluster)  [unwired: 10 in]
        n133 = Merge Errors(w484, w500, w496) -> (w485:errorcluster)
      }
      frame "---Copy This Frame---" {
        # "Duplicate this frame when creating new messages.  Change this comment in the duplicated frame to describe this message."
        n134 = Merge Errors(w505) -> (w504:errorcluster)
      }
      frame Default {
        # "'Default' case only runs if there is a message that isn't defined in any of the other cases.  Output a programming error."
        n135 = xnode "Error Ring"("parameter 0"=w507) -> ("error out"=w506:errorcluster)
      }
    }
    n136 = call "CML Error Handler - Message Handling Loop.vi"("error in (no error)"=w278, "Message Queue"=w277) -> ("dup error in"=w279:errorcluster)  [unwired: 8 in, 1 out]
  }
  n137 = while {
    tunnel: [w522] -> w21
    shift-right: [w524] -> w17
    shift-left: w9 -> [w525]
    tunnel: w1 -> [w519]
    stop <- w523 stop-if-true
    # "Event Handling Loop"
    n138 = Unbundle By Name(w519) -> ("UI"=w518:refnum<queue>)
    n139 = event shown="[1] \"Settings\": Value Change" {
      selector: w525 -> [_ _ _ _ _ _ _]
      dyn-events: [_ _ _ _ _ _ _] -> w524
      timeout: _ -> [_ _ _ _ _ _ _]
      tunnel: [_ _ _ _ _ _ TRUE ("Discard?")] -> w523
      tunnel: [w529 w532 w537 w541 _ w549 _] -> w521
      tunnel: [w528 w533 w536 w542 w544 w547 w550] -> w520
      tunnel: w518 -> [w527 w531 w535 w539 w544 w546 w550]
      event "Start": Value Change {
        n140 = event-data() -> ()  [unwired: 1 in, 1 out]
        n141 = call-poly "Enqueue Message.vi"("Message"="Start", "Message Queue"=w527) -> ("error out"=w529:errorcluster, "dup Message Queue"=w528:refnum<queue>)  [unwired: 8 in]
      }
      event "Settings": Value Change {
        n142 = event-data() -> ()  [unwired: 1 in, 1 out]
        n143 = call-poly "Enqueue Message.vi"("Message"="Launch Settings Dialog", "Message Queue"=w531) -> ("error out"=w532:errorcluster, "dup Message Queue"=w533:refnum<queue>)  [unwired: 8 in]
      }
      event "Stop": Value Change {
        n144 = event-data() -> ()  [unwired: 1 in, 1 out]
        n145 = call-poly "Enqueue Message.vi"("Message"="Stop", "Message Queue"=w535) -> ("error out"=w537:errorcluster, "dup Message Queue"=w536:refnum<queue>)  [unwired: 8 in]
      }
      event Panel Close? {
        # "Send the 'Confirm Quit' message if the user closes the panel of the VI. Discard the event so the 'Confirm Quit' message has a chance to run."
        n146 = event-data() -> ()  [unwired: 1 in, 1 out]
        n147 = call-poly "Enqueue Message.vi"("Priority Message? (F)"=TRUE, "Message"="Confirm Quit", "Message Queue"=w539) -> ("error out"=w541:errorcluster, "dup Message Queue"=w542:refnum<queue>)  [unwired: 7 in]
        n148 = event-data("Discard?"=TRUE) -> ()  [unwired: 1 in, 1 out]
      }
      event Application Instance Close {
        n149 = event-data() -> ()  [unwired: 1 in, 1 out]
      }
      event "Exit": Value Change {
        w548 = TRUE  # Priority Message
        # "The UI Message Loop handles sending the Exit message to other loops."
        n150 = event-data() -> ()  [unwired: 1 in, 1 out]
        n151 = call-poly "Enqueue Message.vi"("Priority Message? (F)"=w548, "Message"="Exit", "Message Queue"=w546) -> ("error out"=w549:errorcluster, "dup Message Queue"=w547:refnum<queue>)  [unwired: 7 in]
      }
      event User Event {
        # "The Message Handling Loop processed an \"Exit\" message, which fired this event to stop the Event Handling Loop."
        n152 = event-data() -> ()  [unwired: 1 in, 1 out]
        n153 = local write "Status"("Exit" ("Exit String")) -> ()
      }
    }
    n154 = call "CML Error Handler - Event Handling Loop.vi"("error in (no error)"=w521, "Message Queue"=w520) -> ("dup error in"=w522:errorcluster)  [unwired: 8 in, 1 out]
  }
  n155 = Unregister For Events(event registration refnum=w17, error in=w21) -> (error out=w18:errorcluster)
  n156 = Release Queue(queue=w22, error in (no error)=w23) -> (error out=w12:errorcluster)  [unwired: 1 in, 2 out]
  n157 = Release Notifier(notifier=w5, error in (no error)=w12) -> (error out=w11:errorcluster)  [unwired: 1 in, 2 out]
  n158 = Merge Errors(w18, w11, w4, w2) -> (w14:errorcluster)
  n159 = call "Destroy User Event - Stop.vi"("error in (no error)"=w14, "User Event - Stop"=w8) -> ("error out"=w13:errorcluster)  [unwired: 9 in]
  n160 = disable-structure shown="RUN_TIME_ENGINE==True" {
    disable-tunnel: w13 -> [_ _]
    frame condition #0 (active) {
    }
    frame condition #1 {
      # "Call Quit LabVIEW if running as a built application."
      n161 = Quit LabVIEW() -> ()  [unwired: 1 in]
    }
  }
